vi "testDBConnection.vi"() -> ()   [LabVIEW 2018]
uses:
  <vilib>/addons/database/Connection.llb/DB Tools Open Connec (Path).vi
  <vilib>/addons/database/NI_Database_API.lvlib
panel:
  out "data 2":string[][](array[string])
  out "error out 2":errorcluster
  in  "error out":errorcluster
  out "tables":string[](array[string])
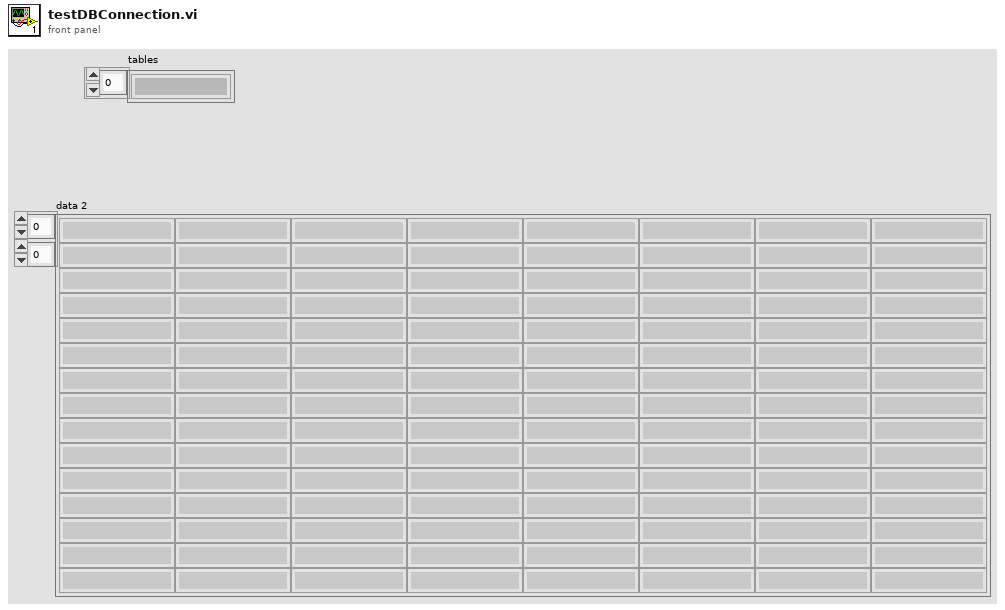
[diagram p1: front panel]
types:
  T1 = typedef "NI_Database_API.lvlib/Conn ObjectReference.ctl" = refnum<k1>
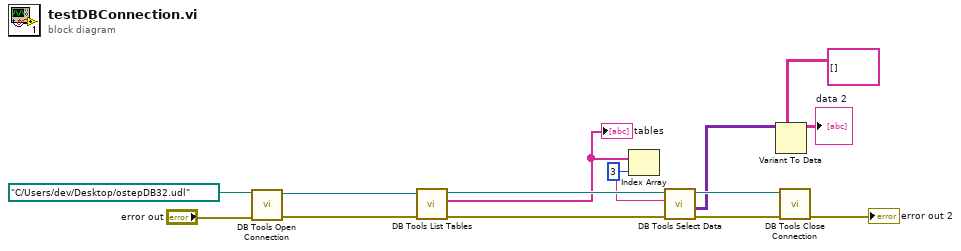
[diagram p0: block diagram]
diagram:
  n1 = call-poly <vilib>:"DB Tools Open Connection.vi"("error in (no error)"="error out", "connection information"=path "C:/Users/dev/Desktop/ostepDB32.udl") -> ("error out"=w14:errorcluster, "connection reference"=w15:T1)  [unwired: 6 in]
  n2 = call <vilib>:"DB Tools List Tables.vi"("error in (no error)"=w14, "connection reference"=w15) -> ("error out"=w12:errorcluster, "tables"=w9:string[], "connection reference out"=w13:T1)  [unwired: 3 in]
  "tables" <- w9
  n3 = Index Array(array=w9, index=3) -> (element=w7:string)
  n4 = call <vilib>:"DB Tools Select Data.vi"("error in (no error)"=w12, "table"=w7, "connection reference"=w13) -> ("error out"=w11:errorcluster, "data"=w3:variant[][], "connection reference out"=w10:T1)  [unwired: 3 in]
  n5 = Variant To Data(type=string[][] [], Variant=w3) -> (data=→"data 2":string[][])  [unwired: 1 in, 1 out]
  n6 = call <vilib>:"DB Tools Close Connection.vi"("error in (no error)"=w11, "connection reference"=w10) -> ("error out"=→"error out 2":errorcluster)  [unwired: 5 in]
